vi "Launch Tasks.vi"(7 "Core APIs":T1, 8 "error in (no error)":errorcluster, 11 "DemoApp in":refnum<class "DemoApp.lvclass">) -> (0 "error out":errorcluster, 3 "DemoApp out":refnum<class "DemoApp.lvclass">)   [LabVIEW 2020, in "VolatusDemo.lvlib" / "DemoApp.lvclass"]
uses:
  DemoApp.lvclass
  DemoApp.lvclass/DemoApp.ctl
  VolatusDataLogger/LoggingManager/LoggingManager.lvclass
  Volatus/VolatusAPI/VolatusAPI.lvclass
  Volatus/Event API/EventAPI.lvclass
  Volatus/TelemetryAPI/TelemetryAPI.lvclass
  Volatus/Core APIs.ctl
  Volatus/Volatus.lvlib
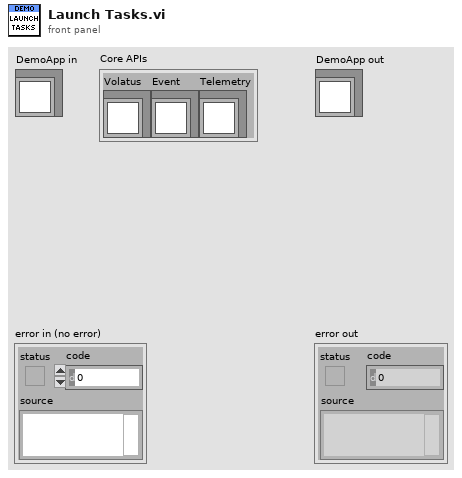
[diagram p1: front panel]
types:
  T1 = typedef "Volatus.lvlib/Core APIs.ctl" = cluster{"Volatus":refnum<class "VolatusAPI.lvclass">, "Event":refnum<class "EventAPI.lvclass">, "Telemetry":refnum<class "TelemetryAPI.lvclass">}
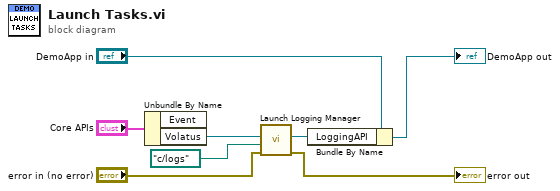
[diagram p0: block diagram]
diagram:
  n1 = Unbundle By Name("Core APIs") -> ("Volatus"=w7:refnum<class "VolatusAPI.lvclass">)  [unwired: 1 out]
  n2 = call "Launch Logging Manager.vi"("error in (no error)"="error in (no error)", "Logging Root"=path "c:/logs", "VolatusAPI"=w7) -> ("error out"=→"error out":errorcluster, "LoggingAPI"=w3:refnum<class "LoggingAPI.lvclass">)  [unwired: 7 in]
  n3 = Bundle By Name(cluster="DemoApp in", "LoggingAPI"=w3) -> (→"DemoApp out":refnum<class "DemoApp.lvclass">)
